vi "RecVOR.vi"() -> ()   [LabVIEW 2013]
uses:
  <vilib>/userdefined/High Color/IMAQdx.ctl
  <vilib>/vision/Avi1.llb/AviRefnum.ctl
  <vilib>/vision/driver/IMAQdx.llb/IMAQdx Attribute Visibility.ctl
  <vilib>/Instr/_visa.llb/VISA Configure Serial Port (Instr).vi
  <vilib>/DAQmx/read.llb/DAQmx Read (Digital Bool 1Line 1Point).vi
  <vilib>/DAQmx/read.llb/DAQmx Read (Counter U32 1Chan 1Samp).vi
  <vilib>/Utility/file.llb/Write To Spreadsheet File (DBL).vi
  <vilib>/vision/driver/NI_Vision_Acquisition_Software.lvlib
  <resource>/objmgr/imaqdx.rc
  <vilib>/vision/NI_Vision_Development_Module.lvlib
panel:
  out "NewRecevie":string
  in  "Use":bool=TRUE
  out "Serial 2":bool
  out "Serial":bool
  in  "Tilting":refnum<visa-resource-name>="COM4"
  in  "Image Flip":u32(ring) items=["Horizontal Flip", "Vertical Flip", "Central Flip", "No Flip"]
  in  "Attribute Name":u32(ring)
  in  "Set":bool
  in  "Attribute Value":string
  in  "Arduino":refnum<visa-resource-name>="COM6"
  out "Pos./Vel.":cluster{dbl, dbl}(graph)
  out "Start RecTime":timestamp
  out "Avi Refnum":T1
  out "Elapsed Time":dbl
  out "Frame Num":dbl
  in  "Codec:":string(combo)="Microsoft Video 1"
  out "Rec File Path:":path
  in  "Recording":bool
  in  "Camera Name:":T2="cam1"
  in  "stop":bool
  in  "OpenCam":bool
  out "Frame Rate":dbl(knob) scale=0.0..120.0
  in  "Tab Control":enum32{"Alignment", "Rotator"}(tab)
  out "Alignment":bool
  in  "BCGT":T3={"Brightness"=171.0, "Contrast"=89.0, "Gamma"=2.0, "Threshold_Low"=0.0, "Threshold_High"=255.0} {"Threshold_High" min=0.0 max=255.0 step=1.0 scale=0.0..255.0; "Threshold_Low" min=0 max=255 step=1 scale=0.0..255.0 scale format="%.2f"; "Gamma" min=0.1 max=10 step=0.01 scale=0.1..10.0 scale format="%.1f"; "Contrast" min=1 max=89 step=0.1 scale=0.0..89.0 scale format="%.2f"; "Brightness" min=0 max=255 step=1 scale=0.0..255.0 scale format="%.2f"}
  out "Number of Particles":i32
  out "Distances":sgl[](array[numeric]) format="%.4f"
  out "Array":cluster{"Numeric":dbl, "Numeric":dbl}[](array[cluster])
  out "Image 2":T4(plugin-control)
  in  "primary":bool
  in  "Clear 2":bool
  in  "Clear":bool
  in  "Tolerence":dbl=90.0
  in  "Add":bool
  in  "mode":enum32{"Sine", "Linear", "Tilting"}(tab)
  in  "Freq":string="0.01" caption="Freq.(Hz)"
  in  "Time":string="10" caption="Operation \nTime(sec)"
  in  "Ang.vel":string="30" caption="Angular\nVelocity\n( ˚/sec)"
  in  "IncT":string="2000" caption="Acceleration\n( ˚/sec²)"
  in  "Ang.vel 2":string="100" caption="Angular\nVelocity\n( ˚/sec)"
  in  "Time 2":string="10" caption="Operation Time(sec)"
  in  "Direction":enum32{"Radio Selection 1", "Radio Selection 2"}(radio)
  out "TiltingLED":bool
  in  "TilAngle":string="30" caption="Tilting\nAngle"
  in  "TilTime":string="2" caption="Tilting\nTime"
  out "ObjAng":dbl
  out "TiltAng.":dbl
  out "WMode":enum16{"stop", "goFront", "goBack"}(ring)
  in  "SeeAngle":bool
  out "check":bool
  out "Degree/sec":dbl(knob) scale=-105.0..105.0
  out "EMST":bool
  out "SVON":bool=TRUE
  out "Received Data":string
  out "Transmit Data":string
  in  "Sent":bool
  in  "task/channels in":refnum<k21>="position"
  in  "task/channels in 2":refnum<k21>="dir"
  in  "task/channels in 3":refnum<k21>="dir_vel"
  out "Angle Position":dbl(knob)
  out "List":string
  in  "StopT":bool
  out "Image":T4(plugin-control)
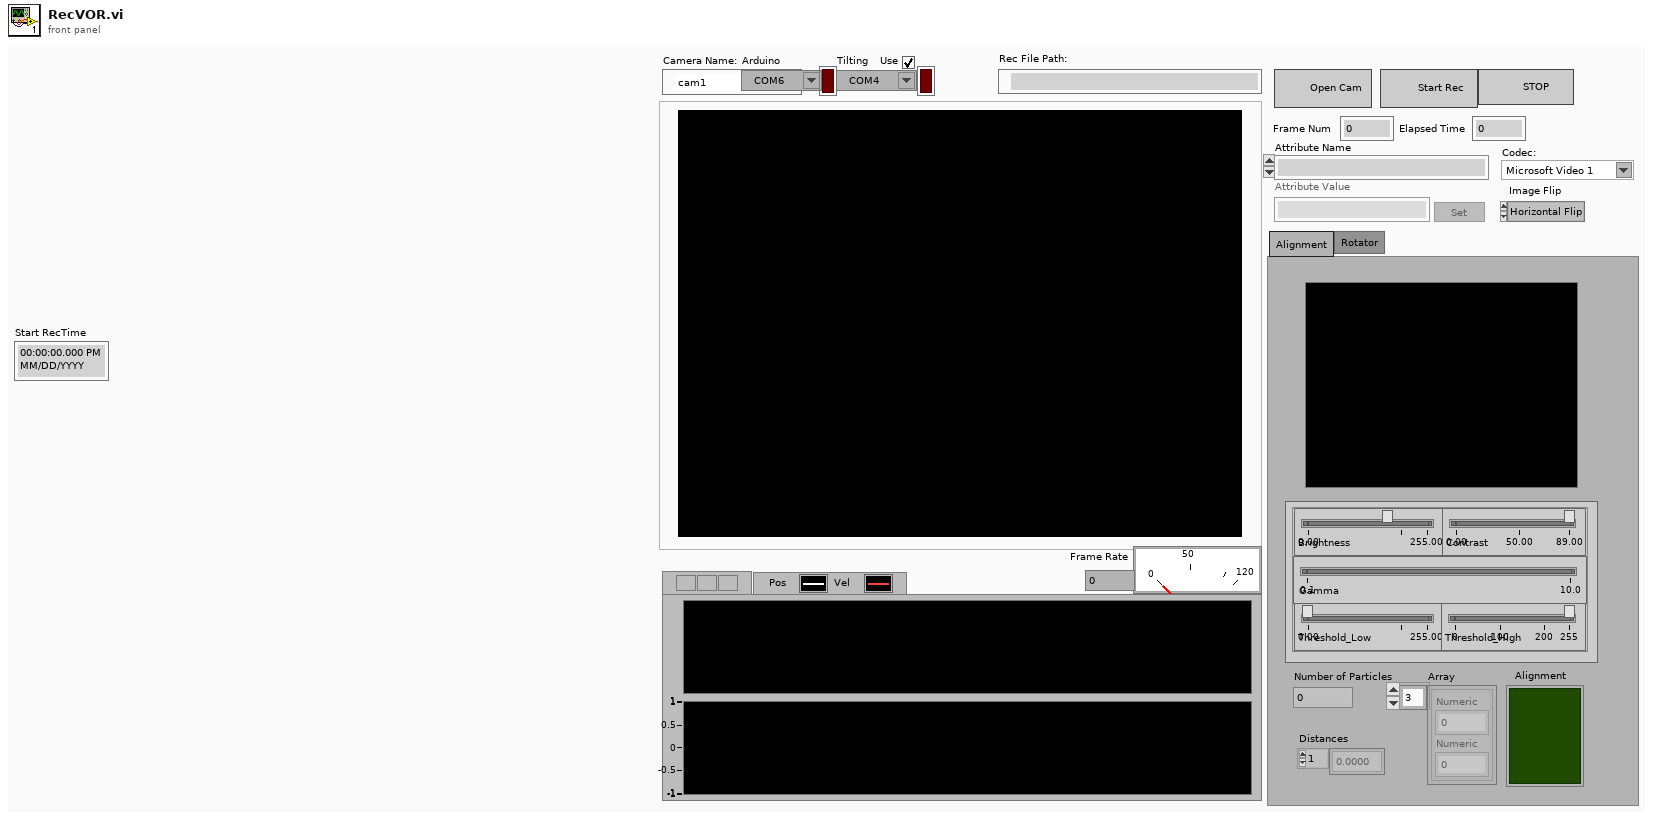
[diagram p1: front panel]
types:
  T1 = typedef "AviRefnum.ctl" = refnum<k1>
  T2 = typedef "IMAQdx.ctl" = refnum<k21>
  T3 = cluster{"Brightness":sgl, "Contrast":sgl, "Gamma":sgl, "Threshold_Low":sgl, "Threshold_High":dbl}
  T4 = typedef "IMAQ Image.ctl" = refnum<image>
  T5 = enum8{"Enabled", "Disabled", "Disabled and Grayed Out"}
  T6 = enum16{"Calvar3Open", "CalDataOpen", "CalGrpOpen", "AddAvg", "RmvAvg", "CalCalvar", "AddVar", "SaveVar", "Up", "Dn", "Del"}
  T7 = enum16{"SVON OFF", "SVON ON", "EMST OFF", "EMST ON", "15 degree, 0.1Hz", "15 degree, 0.2Hz", "15 degree, 0.5Hz", "15 degree, 1Hz", "15 degree, 2Hz", "15 degree, 4Hz", "15 degree, 6Hz", "15 degree, 8Hz", "15 degree, 10Hz", "30 degree, 0.1Hz", "30 degree, 0.2Hz", "30 degree, 0.5Hz", "30 degree, 1Hz", "30 degree, 2Hz", "30 degree, 4Hz", "30 degree, 6Hz", "30 degree, 8Hz", "30 degree, 10Hz", "60 degree, 0.1Hz", "60 degree, 0.2Hz", "60 degree, 0.5Hz", "60 degree, 1Hz", "60 degree, 2Hz", "60 degree, 4Hz", "60 degree, 6Hz", "60 degree, 8Hz", "100 degree, 0.1Hz", "100 degree, 0.2Hz", "100 degree, 0.5Hz", "100 degree, 1Hz"}
  T8 = typedef "NI_Vision_Acquisition_Software.lvlib/IMAQdx Attribute Visibility.ctl" = enum32{"Simple", "Intermediate", "Advanced"}
  T9 = typedef "NI_Vision_Acquisition_Software.lvlib/IMAQdx Attribute Type.ctl" = enum32{"U32", "I64", "DBL", "String", "Enum", "Bool", "Command"}
  T10 = cluster{"Attribute Type":T9, "Readable":bool, "Writable":bool, "Attribute Name":string}[]
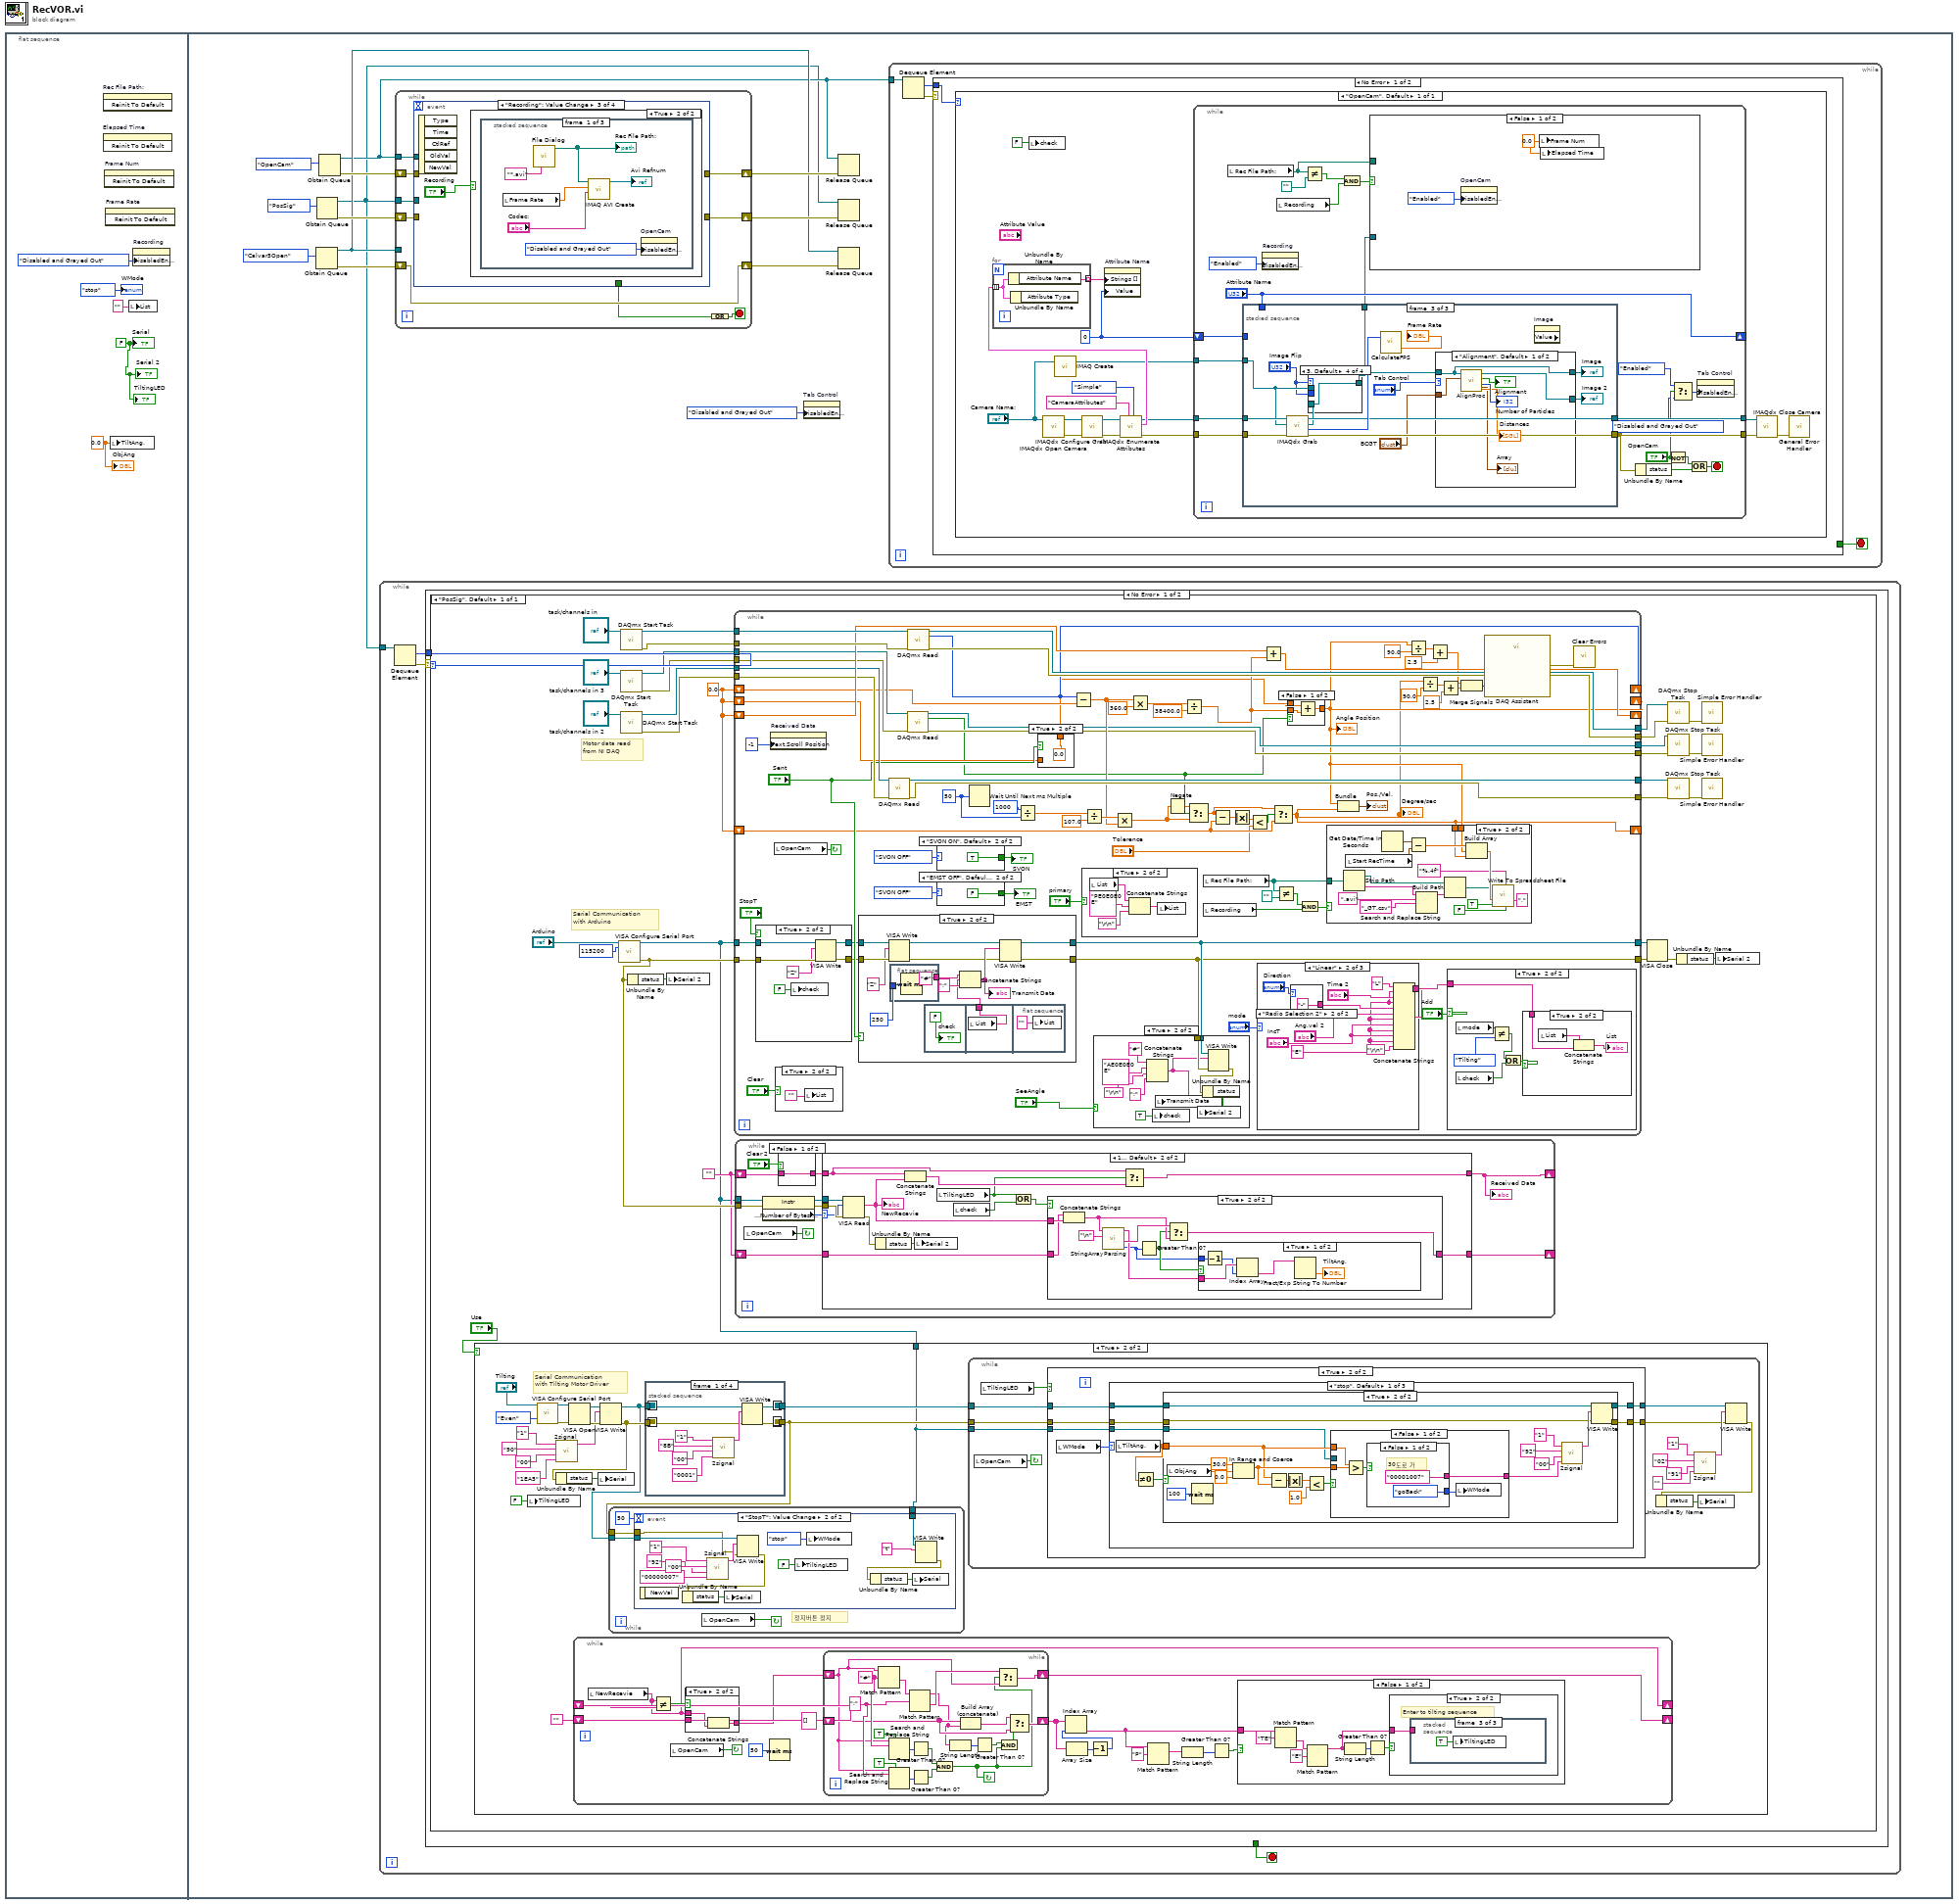
[diagram p0: block diagram]
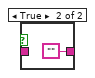
[diagram p2: hidden frame]
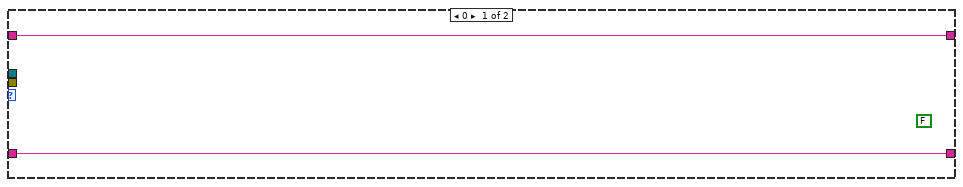
[diagram p3: hidden frame]
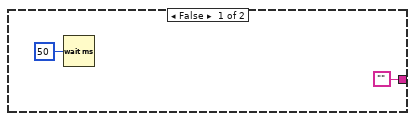
[diagram p4: hidden frame]
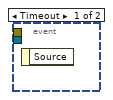
[diagram p7: hidden frame]
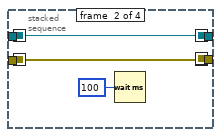
[diagram p8: hidden frame]
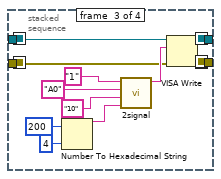
[diagram p9: hidden frame]
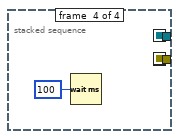
[diagram p10: hidden frame]
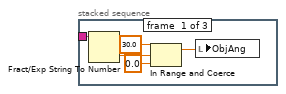
[diagram p12: hidden frame]
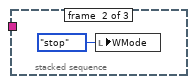
[diagram p13: hidden frame]
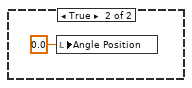
[diagram p14: hidden frame]
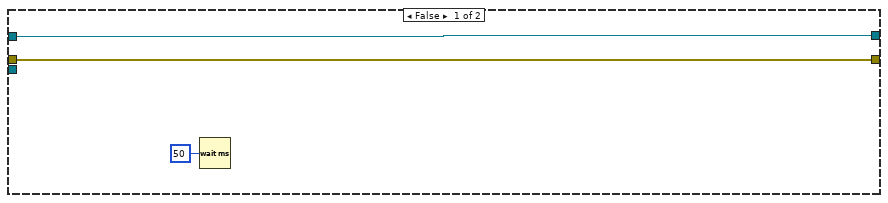
[diagram p16: hidden frame]
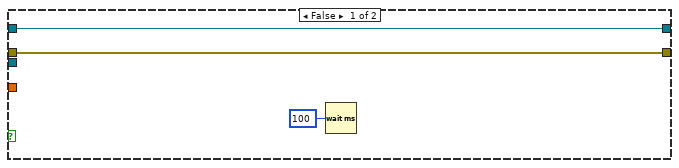
[diagram p17: hidden frame]
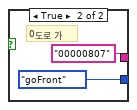
[diagram p18: hidden frame]
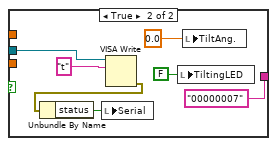
[diagram p19: hidden frame]
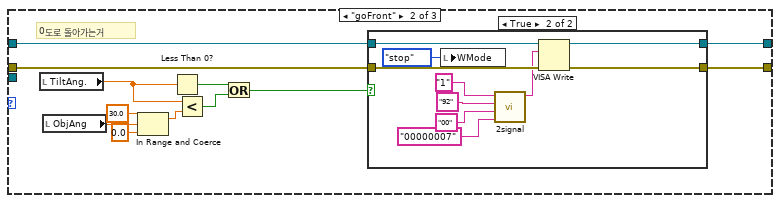
[diagram p20: hidden frame]
diagram:
  n1 = flat-sequence {
    frame #0 {
      w3 = 0.0 ("element")
      w2 = FALSE ("Serial")
      n2 = invoke on="Rec File Path:" class="Path" method="Reinit To Default"() -> ()  [unwired: 3 in, 3 out]
      n3 = invoke on="Elapsed Time" class="DigNum (strict)" method="Reinit To Default"() -> ()  [unwired: 3 in, 3 out]
      n4 = invoke on="Frame Num" class="DigNum (strict)" method="Reinit To Default"() -> ()  [unwired: 3 in, 3 out]
      n5 = invoke on="Frame Rate" class="Knob (strict)" method="Reinit To Default"() -> ()  [unwired: 3 in, 3 out]
      n6 = local write "TiltAng."(w3) -> ()
      n7 = local write "List"("" ("List")) -> ()
      n8 = property on="Recording" class="Bool (strict)"("DisabledEnum"=T5."Disabled and Grayed Out" ("Disabled")) -> ()  [unwired: 2 in, 2 out]
      "Serial" <- w2
      "Serial 2" <- w2
      "ObjAng" <- w3
      "TiltingLED" <- w2
      "WMode" <- enum16{"stop", "goFront", "goBack"}."stop" ("WMode")
    }
    frame #1 {
      n9 = Obtain Queue(element data type=T6."Calvar3Open" ("Enum")) -> (queue out=w9:refnum<queue>, error out=w14:errorcluster)  [unwired: 4 in, 1 out]
      n10 = Obtain Queue(element data type=enum16{"PosSig"}."PosSig" ("Enum")) -> (queue out=w7:refnum<queue>, error out=w15:errorcluster)  [unwired: 4 in, 1 out]
      n11 = Obtain Queue(element data type=enum16{"OpenCam"}."OpenCam" ("Enum")) -> (queue out=w8:refnum<queue>, error out=w17:errorcluster)  [unwired: 4 in, 1 out]
      n12 = while {
        tunnel: w7 -> [w22]
        stop <- w20 stop-if-true
        n13 = Dequeue Element(queue=w22) -> (element=w19:enum16{"PosSig"}, error out=w21:errorcluster)  [unwired: 2 in, 2 out]
        n14 = case shown="No Error" w21 {
          tunnel: [_ TRUE] -> w20
          tunnel: w19 -> [w23 _]
          frame No Error {
            n15 = case shown="\"PosSig\", Default" w23 {
              frame "PosSig", Default {
                w29 = 0.0 ("data")
                w25 = ""
                # "Motor data read\nfrom NI DAQ"
                # "Serial Communication \nwith Arduino"
                n16 = call-poly "VISA Configure Serial Port"("VISA resource name"="Arduino", "baud rate (9600)"=u32 115200) -> ("VISA resource name out"=w24:refnum<visa-resource-name>, "error out"=w28:errorcluster)  [unwired: 12 in]
                n17 = case shown="True" "Use" {
                  tunnel: w24 -> [_ w100]
                  frame False {
                  }
                  frame True {
                    w104 = ""
                    # "Serial Communication\nwith Tilting Motor Driver"
                    n18 = local write "TiltingLED"(FALSE ("TiltingLED")) -> ()
                    n19 = call-poly "VISA Configure Serial Port"("VISA resource name"="Tilting", "parity (0:none)"=enum16{"None", "Odd", "Even", "Mark", "Space"}."Even") -> ("VISA resource name out"=w108:refnum<visa-resource-name>, "error out"=w110:errorcluster)  [unwired: 12 in]
                    n20 = call "2signal.vi"("데이터"="1EA5", "Dat.Num"="00", "커맨드"="90", "국번"="1") -> ("String"=w107:string)  [unwired: 7 in]
                    n21 = VISA Open(error in (no error)=w110, VISA resource name=w108) -> (VISA resource name=w113:refnum<visa-resource-name>, error out=w112:errorcluster)  [unwired: 3 in]
                    n22 = while {
                      shift-right: [w175] -> _
                      shift-left: w104 -> [w176]
                      shift-right: [w170] -> _
                      shift-left: w104 -> [w172]
                      stop <- w173 continue-if-true
                      n23 = local read "NewRecevie"() -> (w170:string)
                      n24 = Not Equal?(x=w170, y=w172) -> (x != y?=w171:bool)
                      n25 = local read "OpenCam"() -> (w173:bool)
                      n26 = case shown="True" w171 {
                        tunnel: w176 -> [w218 w221]
                        tunnel: [w218 w220] -> w180
                        tunnel: w170 -> [_ w219]
                        frame False {
                        }
                        frame True {
                          n27 = Concatenate Strings(w221, w219) -> (w220:string)
                        }
                      }
                      n28 = Wait (ms)(milliseconds to wait=u32 50) -> ()  [unwired: 1 out]
                      n29 = while {
                        shift-right: [w205] -> w177
                        shift-left: string[] [] -> [w203]
                        shift-right: [w208] -> w175
                        shift-left: w180 -> [w206]
                        stop <- w199 continue-if-true
                        w213 = ";" ("regular expression")
                        w215 = "#" ("regular expression")
                        n30 = Match Pattern(string=w206, regular expression=w215) -> (after substring=w217:string)  [unwired: 1 in, 3 out]
                        n31 = Search and Replace String(replace all?=TRUE ("replace all? (F)"), input string=w206, search string=w215) -> (number of replacements=w212:i32)  [unwired: 5 in, 3 out]
                        n32 = Search and Replace String(replace all?=TRUE ("replace all? (F)"), input string=w206, search string=w213) -> (number of replacements=w211:i32)  [unwired: 5 in, 3 out]
                        n33 = Match Pattern(string=w217, regular expression=w213) -> (before substring=w202:string, after substring=w207:string)  [unwired: 1 in, 2 out]
                        n34 = Greater Than 0?(x=w212) -> (x > 0?=w209:bool)
                        n35 = Greater Than 0?(x=w211) -> (x > 0?=w210:bool)
                        n36 = And(x=w209, y=w210) -> (x .and. y?=w199:bool)
                        n37 = String Length(string=w202) -> (length=w201:i32)
                        n38 = Build Array (concatenate)(w203, w202) -> (w204:string[])
                        n39 = Greater Than 0?(x=w201) -> (x > 0?=w200:bool)
                        n40 = Select(t=w207, s=w199, f=w206) -> (s? t:f=w208:string)
                        n41 = And(x=w200, y=w199) -> (x .and. y?=w198:bool)
                        n42 = Select(t=w204, s=w198, f=w203) -> (s? t:f=w205:string[])
                      }
                      n43 = Array Size(array=w177) -> (size(s)=w178:i32)
                      n44 = Decrement(x=w178) -> (x-1=w179:i32)
                      n45 = Index Array(array=w177, index=w179) -> (element=w168:string)
                      n46 = Match Pattern(string=w168, regular expression="P") -> (match substring=w165:string)  [unwired: 1 in, 3 out]
                      n47 = String Length(string=w165) -> (length=w167:i32)
                      n48 = Greater Than 0?(x=w167) -> (x > 0?=w166:bool)
                      n49 = case shown="False" w166 {
                        tunnel: w168 -> [w188 _]
                        frame False {
                          n50 = Match Pattern(string=w188, regular expression="TE") -> (after substring=w185:string)  [unwired: 1 in, 3 out]
                          n51 = Match Pattern(string=w185, regular expression="E") -> (before substring=w182:string)  [unwired: 1 in, 3 out]
                          n52 = String Length(string=w182) -> (length=w184:i32)
                          n53 = Greater Than 0?(x=w184) -> (x > 0?=w183:bool)
                          n54 = case shown="True" w183 {
                            tunnel: w182 -> [_ w189]
                            frame False {
                            }
                            frame True {
                              # "Enter to tilting sequence"
                              n55 = stacked-sequence {
                                tunnel: w189 -> [w194 _ _]
                                frame #0 {
                                n56 = Fract/Exp String To Number(string=w194) -> (number=w193:dbl)  [unwired: 3 in, 1 out]
                                n57 = In Range and Coerce(upper limit=30.0, x=w193, lower limit=0.0) -> (coerced(x)=w192:dbl)  [unwired: 1 out]
                                n58 = local write "ObjAng"(w192) -> ()
                                }
                                frame #1 {
                                n59 = local write "WMode"(enum16{"stop", "goFront", "goBack"}."stop" ("WMode")) -> ()
                                }
                                frame #2 {
                                n60 = local write "TiltingLED"(TRUE ("TiltingLED")) -> ()
                                }
                              }
                            }
                          }
                        }
                        frame True {
                          n61 = local write "Angle Position"(0.0 ("Angle Position")) -> ()
                        }
                      }
                    }
                    n62 = VISA Write(VISA resource name=w113, write buffer=w107, error in (no error)=w112) -> (VISA resource name out=w102:refnum<visa-resource-name>, error out=w106:errorcluster)  [unwired: 1 out]
                    n63 = Unbundle By Name(w106) -> ("status"=w118:bool)
                    n64 = local write "Serial"(w118) -> ()
                    n65 = stacked-sequence {
                      seq-local: [w140 _ _ _] -> [_ w149 _ _]
                      seq-local: [w139 _ _ _] -> [_ w148 _ _]
                      seq-local: [_ w149 _ _] -> [_ _ w155 _]
                      seq-local: [_ w148 _ _] -> [_ _ w154 _]
                      seq-local: [_ _ w152 _] -> [_ _ _ w163]
                      seq-local: [_ _ w151 _] -> [_ _ _ w162]
                      tunnel: w102 -> [w142 _ _ _]
                      tunnel: w106 -> [w141 _ _ _]
                      tunnel: [_ _ _ w163] -> w105
                      tunnel: [_ _ _ w162] -> w101
                      frame #0 {
                        n66 = call "2signal.vi"("데이터"="0001", "Dat.Num"="00", "커맨드"="8B", "국번"="1") -> ("String"=w143:string)  [unwired: 7 in]
                        n67 = VISA Write(VISA resource name=w142, write buffer=w143, error in (no error)=w141) -> (VISA resource name out=w140:refnum<visa-resource-name>, error out=w139:errorcluster)  [unwired: 1 out]
                      }
                      frame #1 {
                        n68 = Wait (ms)(milliseconds to wait=u32 100) -> ()  [unwired: 1 out]
                      }
                      frame #2 {
                        n69 = Number To Hexadecimal String(1:i16 4 ("width (-)"), 2:200 ("number")) -> (0:w156:string)
                        n70 = call "2signal.vi"("데이터"=w156, "Dat.Num"="10", "커맨드"="A0", "국번"="1") -> ("String"=w161:string)  [unwired: 7 in]
                        n71 = VISA Write(VISA resource name=w155, write buffer=w161, error in (no error)=w154) -> (VISA resource name out=w152:refnum<visa-resource-name>, error out=w151:errorcluster)  [unwired: 1 out]
                      }
                      frame #3 {
                        n72 = Wait (ms)(milliseconds to wait=u32 100) -> ()  [unwired: 1 out]
                      }
                    }
                    n73 = while {
                      tunnel: w102 -> [w122]
                      tunnel: w101 -> [w121]
                      tunnel: w100 -> [w119]
                      stop <- w120 continue-if-true
                      # "정지버튼 정지"
                      n74 = event shown="[1] \"StopT\": Value Change" {
                        selector: _ -> [_ _]
                        dyn-events: _ -> [_ _]
                        timeout: 50 -> [_ _]
                        tunnel: w122 -> [_ w131]
                        tunnel: w121 -> [_ w130]
                        tunnel: w119 -> [_ w124]
                        event Timeout {
                          n75 = event-data() -> ()  [unwired: 1 in, 1 out]
                        }
                        event "StopT": Value Change {
                          n76 = event-data() -> ()  [unwired: 1 in, 1 out]
                          n77 = call "2signal.vi"("데이터"="00000007", "Dat.Num"="00", "커맨드"="92", "국번"="1") -> ("String"=w134:string)  [unwired: 7 in]
                          n78 = VISA Write(VISA resource name=w131, write buffer=w134, error in (no error)=w130) -> (error out=w132:errorcluster)  [unwired: 2 out]
                          n79 = Unbundle By Name(w132) -> ("status"=w133:bool)
                          n80 = local write "Serial"(w133) -> ()
                          n81 = local write "TiltingLED"(FALSE ("TiltingLED")) -> ()
                          n82 = local write "WMode"(enum16{"stop", "goFront", "goBack"}."stop" ("WMode")) -> ()
                          n83 = VISA Write(VISA resource name=w124, write buffer="t") -> (error out=w125:errorcluster)  [unwired: 1 in, 2 out]
                          n84 = Unbundle By Name(w125) -> ("status"=w127:bool)
                          n85 = local write "Serial"(w127) -> ()
                        }
                      }
                      n86 = local read "OpenCam"() -> (w120:bool)
                    }
                    n87 = while {
                      tunnel: w105 -> [w226]
                      tunnel: w101 -> [w223]
                      tunnel: w100 -> [w222]
                      stop <- w235 continue-if-true
                      n88 = local read "OpenCam"() -> (w235:bool)
                      n89 = local read "TiltingLED"() -> (w227:bool)
                      n90 = case shown="True" w227 {
                        tunnel: w226 -> [w238 w244]
                        tunnel: w223 -> [w237 w243]
                        tunnel: [w238 w242] -> w229
                        tunnel: [w237 w241] -> w228
                        tunnel: w222 -> [_ w239]
                        frame False {
                          n91 = Wait (ms)(milliseconds to wait=u32 50) -> ()  [unwired: 1 out]
                        }
                        frame True {
                          n92 = local read "WMode"() -> (w240:enum16{"stop", "goFront", "goBack"})
                          n93 = case shown="\"stop\", Default" w240 {
                            tunnel: w244 -> [w251 w302 w326]
                            tunnel: w243 -> [w250 w301 w325]
                            tunnel: [w248 w299 w323] -> w242
                            tunnel: [w249 w300 w324] -> w241
                            tunnel: w239 -> [w247 _ _]
                            frame "stop", Default {
                              n94 = local read "TiltAng."() -> (w246:dbl)
                              n95 = Not Equal To 0?(x=w246) -> (x != 0?=w245:bool)
                              n96 = case shown="True" w245 {
                                tunnel: w251 -> [w254 w271]
                                tunnel: w250 -> [w253 w270]
                                tunnel: [w253 w268] -> w249
                                tunnel: [w254 w267] -> w248
                                tunnel: w246 -> [_ w257]
                                tunnel: w247 -> [_ w255]
                                frame False {
                                n97 = Wait (ms)(milliseconds to wait=u32 100) -> ()  [unwired: 1 out]
                                }
                                frame True {
                                n98 = local read "ObjAng"() -> (w263:dbl)
                                n99 = Wait (ms)(milliseconds to wait=u32 100) -> ()  [unwired: 1 out]
                                n100 = In Range and Coerce(upper limit=30.0, x=w263, lower limit=0.0) -> (coerced(x)=w261:dbl)  [unwired: 1 out]
                                n101 = Subtract(x=w257, y=w261) -> (x-y=w260:dbl)
                                n102 = Absolute Value(x=w260) -> (abs(x)=w259:dbl)
                                n103 = Less?(x=w259, y=1.0) -> (x < y?=w256:bool)
                                n104 = case shown="False" w256 {
                                tunnel: [w279 "00000007"] -> w266
                                tunnel: w257 -> [w276 _]
                                tunnel: w261 -> [w275 _]
                                tunnel: w255 -> [_ w285]
                                frame False {
                                n105 = Greater?(x=w276, y=w275) -> (0:w277:bool)
                                n106 = case shown="False" w277 {
                                tunnel: ["00001007" "00000807"] -> w279
                                tunnel: [enum16{"stop", "goFront", "goBack"}."goBack" ("WMode") enum16{"stop", "goFront", "goBack"}."goFront" ("WMode")] -> w278
                                frame False {
                                # "30도로 가"
                                }
                                frame True {
                                # "0도로 가"
                                }
                                }
                                n107 = local write "WMode"(w278) -> ()
                                }
                                frame True {
                                n108 = VISA Write(VISA resource name=w285, write buffer="t") -> (error out=w286:errorcluster)  [unwired: 1 in, 2 out]
                                n109 = Unbundle By Name(w286) -> ("status"=w287:bool)
                                n110 = local write "Serial"(w287) -> ()
                                n111 = local write "TiltingLED"(FALSE ("TiltingLED")) -> ()
                                n112 = local write "TiltAng."(0.0 ("lower limit")) -> ()
                                }
                                }
                                n113 = call "2signal.vi"("데이터"=w266, "Dat.Num"="00", "커맨드"="92", "국번"="1") -> ("String"=w272:string)  [unwired: 7 in]
                                n114 = VISA Write(VISA resource name=w271, write buffer=w272, error in (no error)=w270) -> (VISA resource name out=w267:refnum<visa-resource-name>, error out=w268:errorcluster)  [unwired: 1 out]
                                }
                              }
                            }
                            frame "goFront" {
                              # "0도로 돌아가는거"
                              n115 = local read "TiltAng."() -> (w292:dbl)
                              n116 = local read "ObjAng"() -> (w295:dbl)
                              n117 = In Range and Coerce(upper limit=30.0, x=w295, lower limit=0.0) -> (coerced(x)=w294:dbl)  [unwired: 1 out]
                              n118 = Less Than 0?(x=w292) -> (x < 0?=w291:bool)
                              n119 = Less?(x=w292, y=w294) -> (x < y?=w293:bool)
                              n120 = Or(x=w291, y=w293) -> (x .or. y?=w298:bool)
                              n121 = case shown="True" w298 {
                                tunnel: w302 -> [w304 w314]
                                tunnel: w301 -> [w303 w313]
                                tunnel: [w303 w305] -> w300
                                tunnel: [w304 w312] -> w299
                                frame False {
                                }
                                frame True {
                                n122 = local write "WMode"(enum16{"stop", "goFront", "goBack"}."stop" ("WMode")) -> ()
                                n123 = call "2signal.vi"("데이터"="00000007", "Dat.Num"="00", "커맨드"="92", "국번"="1") -> ("String"=w307:string)  [unwired: 7 in]
                                n124 = VISA Write(VISA resource name=w314, write buffer=w307, error in (no error)=w313) -> (VISA resource name out=w312:refnum<visa-resource-name>, error out=w305:errorcluster)  [unwired: 1 out]
                                }
                              }
                            }
                            frame "goBack" {
                              w316 = 30.0 ("upper limit")
                              # "30도로 기울어지는거"
                              n125 = local read "ObjAng"() -> (w320:dbl)
                              n126 = local read "TiltAng."() -> (w317:dbl)
                              n127 = In Range and Coerce(upper limit=w316, x=w320, lower limit=0.0) -> (coerced(x)=w321:dbl)  [unwired: 1 out]
                              n128 = Less?(x=w316, y=w317) -> (x < y?=w315:bool)
                              n129 = Greater?(x=w317, y=w321) -> (0:w322:bool)
                              n130 = Or(x=w315, y=w322) -> (x .or. y?=w318:bool)
                              n131 = case shown="True" w318 {
                                tunnel: w326 -> [w328 w338]
                                tunnel: w325 -> [w327 w337]
                                tunnel: [w327 w336] -> w324
                                tunnel: [w328 w335] -> w323
                                frame False {
                                }
                                frame True {
                                n132 = local write "WMode"(enum16{"stop", "goFront", "goBack"}."stop" ("WMode")) -> ()
                                n133 = call "2signal.vi"("데이터"="00000007", "Dat.Num"="00", "커맨드"="92", "국번"="1") -> ("String"=w330:string)  [unwired: 7 in]
                                n134 = VISA Write(VISA resource name=w338, write buffer=w330, error in (no error)=w337) -> (VISA resource name out=w335:refnum<visa-resource-name>, error out=w336:errorcluster)  [unwired: 1 out]
                                }
                              }
                            }
                          }
                        }
                      }
                      n135 = call "2signal.vi"("데이터"="", "Dat.Num"="91", "커맨드"="02", "국번"="1") -> ("String"=w234:string)  [unwired: 7 in]
                      n136 = VISA Write(VISA resource name=w229, write buffer=w234, error in (no error)=w228) -> (error out=w224:errorcluster)  [unwired: 2 out]
                      n137 = Unbundle By Name(w224) -> ("status"=w225:bool)
                      n138 = local write "Serial"(w225) -> ()
                    }
                  }
                }
                n139 = call <vilib>:"DAQmx Start Task.vi"("task/channels in"="task/channels in") -> ("task out"=w49:refnum<k21>, "error out"=w46:errorcluster)  [unwired: 13 in]
                n140 = call <vilib>:"DAQmx Start Task.vi"("task/channels in"="task/channels in 3") -> ("task out"=w37:refnum<k21>, "error out"=w36:errorcluster)  [unwired: 13 in]
                n141 = call <vilib>:"DAQmx Start Task.vi"("task/channels in"="task/channels in 2") -> ("task out"=w43:refnum<k21>, "error out"=w42:errorcluster)  [unwired: 13 in]
                n142 = Unbundle By Name(w28) -> ("status"=w31:bool)
                n143 = local write "Serial 2"(w31) -> ()
                n144 = while {
                  tunnel: w28 -> [w355]
                  tunnel: w24 -> [w356]
                  tunnel: [w339] -> w52
                  tunnel: [w340] -> w53
                  tunnel: [w411] -> w50
                  tunnel: w49 -> [w410]
                  tunnel: w46 -> [w409]
                  tunnel: [w408] -> w48
                  shift-right: [w399] -> _
                  shift-left: w29 -> [w385]
                  shift-right: [w398] -> _
                  shift-left: w29 -> [w404]
                  tunnel: w43 -> [w403]
                  tunnel: w42 -> [w402]
                  tunnel: [w401] -> w41
                  tunnel: [w400] -> w40
                  shift-right: [w353] -> _
                  shift-left: w29 -> [w384]
                  tunnel: w37 -> [w390]
                  tunnel: w36 -> [w389]
                  tunnel: [w388] -> w34
                  tunnel: [w387] -> w33
                  shift-right: [w347] -> _
                  shift-left: w29 -> [w366]
                  stop <- w362 continue-if-true
                  w397 = u32 50 ("millisecond multiple")
                  n145 = case shown="True" "StopT" {
                    tunnel: [w429 w435] -> w359
                    tunnel: w356 -> [w429 w433]
                    tunnel: [w428 w434] -> w358
                    tunnel: w355 -> [w428 w432]
                    frame False {
                    }
                    frame True {
                      n146 = local write "check"(FALSE ("check")) -> ()
                      n147 = VISA Write(VISA resource name=w433, write buffer="Z", error in (no error)=w432) -> (VISA resource name out=w435:refnum<visa-resource-name>, error out=w434:errorcluster)  [unwired: 1 out]
                    }
                  }
                  n148 = property on="Received Data" class="Str"("Text.Scroll Position"=-1) -> ()  [unwired: 2 in, 2 out]
                  n149 = local read "OpenCam"() -> (w362:bool)
                  n150 = case shown="True" "Clear" {
                    frame False {
                    }
                    frame True {
                      n151 = local write "List"("") -> ()
                    }
                  }
                  n152 = case shown="True" "Sent" {
                    tunnel: w359 -> [w501 w507]
                    tunnel: w358 -> [w500 w506]
                    tunnel: [w501 w513] -> w340
                    tunnel: [w500 w512] -> w339
                    frame False {
                    }
                    frame True {
                      n153 = VISA Write(VISA resource name=w507, write buffer="Z", error in (no error)=w506) -> (VISA resource name out=w504:refnum<visa-resource-name>, error out=w503:errorcluster)  [unwired: 1 out]
                      n154 = flat-sequence {
                        tunnel: ["#"] -> w510
                        tunnel: u32 250 ("millisecond multiple") -> [w514]
                        frame #0 {
                          n155 = Wait (ms)(milliseconds to wait=w514) -> ()  [unwired: 1 out]
                        }
                      }
                      n156 = flat-sequence {
                        tunnel: [w517] -> w508
                        frame #0 {
                          "check" <- FALSE
                        }
                        frame #1 {
                          n157 = local read "List"() -> (w517:string)
                        }
                        frame #2 {
                          n158 = local write "List"("" ("List")) -> ()
                        }
                      }
                      n159 = Concatenate Strings(w510, w508, ";") -> (w509:string)
                      "Transmit Data" <- w509
                      n160 = VISA Write(VISA resource name=w504, write buffer=w509, error in (no error)=w503) -> (VISA resource name out=w513:refnum<visa-resource-name>, error out=w512:errorcluster)  [unwired: 1 out]
                    }
                  }
                  n161 = call-poly <vilib>:"DAQmx Read.vi"("task/channels in"=w403, "error in"=w402) -> ("task out"=w400:refnum<k21>, "error out"=w401:errorcluster)  [unwired: 11 in, 1 out]
                  n162 = call-poly <vilib>:"DAQmx Read.vi"("task/channels in"=w390, "error in"=w389) -> ("task out"=w387:refnum<k21>, "data"=w367:bool, "error out"=w388:errorcluster)  [unwired: 11 in]
                  n163 = call-poly <vilib>:"DAQmx Read.vi"("task/channels in"=w410, "error in"=w409) -> ("task out"=w408:refnum<k21>, "data"=w399:u32, "error out"=w411:errorcluster)  [unwired: 11 in]
                  n164 = case shown="\"SVON ON\", Default" T7."SVON OFF" ("Select Mode") {
                    tunnel: [FALSE TRUE] -> w413
                    frame "SVON OFF" {
                    }
                    frame "SVON ON", Default {
                    }
                  }
                  "SVON" <- w413
                  n165 = case shown="\"EMST OFF\", Default" T7."SVON OFF" ("Select Mode") {
                    tunnel: [TRUE FALSE] -> w412
                    frame "EMST ON" {
                    }
                    frame "EMST OFF", Default {
                    }
                  }
                  "EMST" <- w412
                  n166 = Wait Until Next ms Multiple(millisecond multiple=w397) -> ()  [unwired: 1 out]
                  n167 = Divide(x=u32 1000, y=w397) -> (x/y=w391:dbl)
                  n168 = case shown="True" "Sent" {
                    tunnel: w384 -> [w488 _]
                    tunnel: [w488 0.0] -> w383
                    frame False {
                    }
                    frame True {
                    }
                  }
                  n169 = Subtract(x=w399, y=w385) -> (x-y=w393:dbl)
                  n170 = case shown="True" "primary" {
                    frame False {
                    }
                    frame True {
                      n171 = local read "List"() -> (w425:string)
                      n172 = Concatenate Strings(w425, "PE0E0E0E" ("string"), "\r\n") -> (w424:string)
                      n173 = local write "List"(w424) -> ()
                    }
                  }
                  n174 = Divide(x=w391, y=107.0 ("x")) -> (x/y=w395:dbl)
                  n175 = case shown="True" "SeeAngle" {
                    tunnel: w340 -> [_ w423]
                    tunnel: w339 -> [_ w422]
                    frame False {
                    }
                    frame True {
                      n176 = Concatenate Strings("#", "AE0E0E0E" ("string"), "\r\n", ";") -> (w414:string)
                      n177 = local write "check"(TRUE ("check")) -> ()
                      n178 = local write "Transmit Data"(w414) -> ()
                      n179 = VISA Write(VISA resource name=w423, write buffer=w414, error in (no error)=w422) -> (error out=w420:errorcluster)  [unwired: 2 out]
                      n180 = Unbundle By Name(w420) -> ("status"=w421:bool)
                      n181 = local write "Serial 2"(w421) -> ()
                    }
                  }
                  n182 = Multiply(x=w395, y=w393) -> (x*y=w368:dbl)
                  n183 = Multiply(x=w393, y=360.0) -> (x*y=w406:dbl)
                  n184 = Negate(x=w368) -> (-x=w373:dbl)
                  n185 = Divide(x=w406, y=38400.0) -> (x/y=w394:dbl)
                  n186 = Select(t=w373, s=w367, f=w368) -> (s? t:f=w369:dbl)
                  n187 = local read "Rec File Path:"() -> (w378:path)
                  n188 = local read "Recording"() -> (w361:bool)
                  n189 = Subtract(x=w369, y=w366) -> (x-y=w372:dbl)
                  n190 = Absolute Value(x=w372) -> (abs(x)=w370:dbl)
                  n191 = Less?(x=w370, y="Tolerence") -> (x < y?=w371:bool)
                  n192 = case shown="\"Linear\"" "mode" {
                    tunnel: [w453 w462 w465] -> w363
                    frame "Sine", Default {
                      w447 = "E"
                      n193 = Concatenate Strings("S", w447, "Time", w447, "Ang.vel", w447, "Freq", w447, "\r\n") -> (w453:string)
                    }
                    frame "Linear" {
                      w455 = "E"
                      n194 = case shown="\"Radio Selection 2\"" "Direction" {
                        tunnel: ["" "-"] -> w458
                        frame "Radio Selection 1", Default {
                        }
                        frame "Radio Selection 2" {
                        }
                      }
                      n195 = Concatenate Strings("L", w455, "Time 2", w455, w458, "Ang.vel 2", w455, "IncT", w455, "IncT", w455, "\r\n") -> (w462:string)
                    }
                    frame "Tilting" {
                      w469 = "E"
                      n196 = Concatenate Strings("T", w469, "TilAngle", w469, "TilTime", w469, "\r\n") -> (w465:string)
                    }
                  }
                  n197 = Add(x=w404, y=w394) -> (x+y=w398:dbl)
                  n198 = Select(t=w369, s=w371, f=w366) -> (s? t:f=w347:dbl)
                  "Degree/sec" <- w347
                  n199 = Not Equal?(x=w378, y=path "") -> (x != y?=w380:bool)
                  n200 = case shown="False" w367 {
                    tunnel: w394 -> [w492 w494]
                    tunnel: [w491 w493] -> w353
                    tunnel: w383 -> [w490 w495]
                    frame False {
                      n201 = Add(x=w490, y=w492) -> (x+y=w491:dbl)
                    }
                    frame True {
                      n202 = Subtract(x=w495, y=w494) -> (x-y=w493:dbl)
                    }
                  }
                  "Angle Position" <- w353
                  n203 = And(x=w380, y=w361) -> (x .and. y?=w379:bool)
                  n204 = case shown="True" w379 {
                    tunnel: w353 -> [_ w481]
                    tunnel: w347 -> [_ w480]
                    tunnel: w378 -> [_ w472]
                    frame False {
                    }
                    frame True {
                      n205 = Strip Path(path=w472) -> (stripped path=w474:path, name=w475:string)
                      n206 = local read "Start RecTime"() -> (w487:timestamp)
                      n207 = Get Date/Time In Seconds() -> (seconds since 1Jan1904=w486:timestamp)
                      n208 = Subtract(x=w486, y=w487) -> (x-y=w482:dbl)
                      n209 = Search and Replace String(input string=w475, search string=".avi", replace string="_GT.csv" ("replace string (\"\")")) -> (result string=w478:string)  [unwired: 5 in, 3 out]
                      n210 = Build Path(base path=w474, name or relative path=w478) -> (appended path=w473:path)
                      n211 = Build Array(w482, w481, w480) -> (w479:dbl[])
                      n212 = call-poly <vilib>:"Write To Spreadsheet File.vi"("delimiter (\\t)"="," ("delimiter (\\t)"), "transpose? (no:F)"=FALSE, "format (%.3f)"="%.4f", "append to file? (new file:F)"=TRUE, "1D data"=w479, "file path (dialog if empty)"=w473) -> ()  [unwired: 2 in, 1 out]
                    }
                  }
                  n213 = Bundle(w353, "data"=w347) -> (→"Pos./Vel.":cluster{dbl, "data":dbl})  [unwired: 1 in]
                  n214 = Divide(x=w353, y=90.0) -> (x/y=w351:dbl)
                  n215 = Divide(x=w347, y=90.0) -> (x/y=w349:dbl)
                  n216 = Add(x=w351, y=2.5) -> (x+y=w345:dbl)
                  n217 = Add(x=w349, y=2.5) -> (x+y=w346:dbl)
                  n218 = case shown="True" "Add" {
                    tunnel: w363 -> [_ w437]
                    frame False {
                    }
                    frame True {
                      n219 = local read "mode"() -> (w442:enum32{"Sine", "Linear", "Tilting"})
                      n220 = local read "check"() -> (w440:bool)
                      n221 = Not Equal?(x=w442, y=enum32{"Sine", "Linear", "Tilting"}."Tilting" ("mode")) -> (x != y?=w438:bool)
                      n222 = Or(x=w438, y=w440) -> (x .or. y?=w439:bool)
                      n223 = case shown="True" w439 {
                        tunnel: w437 -> [_ w444]
                        frame False {
                          n224 = One Button Dialog(message="Please check the angle." ("string")) -> ()  [unwired: 1 in, 1 out]
                        }
                        frame True {
                          n225 = local read "List"() -> (w446:string)
                          n226 = Concatenate Strings(w446, w444) -> (→"List":string)
                        }
                      }
                    }
                  }
                  n227 = Merge Signals(w345, w346) -> (w354:dynamicdata)
                  n228 = call "DAQ Assistant"("data"=w354) -> ("error out"=w343:errorcluster)  [unwired: 17 in, 1 out]
                  n229 = call <vilib>:"Clear Errors.vi"("error in (no error)"=w343) -> ()  [unwired: 6 in, 1 out]
                }
                n230 = while {
                  shift-right: [w56] -> _
                  shift-left: w25 -> [w60]
                  tunnel: w24 -> [w59]
                  tunnel: w28 -> [w58]
                  shift-right: [w55] -> _
                  shift-left: w25 -> [w54]
                  stop <- w62 continue-if-true
                  n231 = local read "OpenCam"() -> (w62:bool)
                  n232 = property class="Instr"(reference=w59, error in=w58) -> (reference out=w63:refnum<visa-resource-name>, error out=w64:errorcluster, "Serial Settings:Number of Bytes at Serial Port"=w65:u32)
                  n233 = case shown="False" "Clear 2" {
                    tunnel: w60 -> [w66 _]
                    tunnel: [w66 ""] -> w57
                    frame False {
                    }
                    frame True {
                    }
                  }
                  n234 = case shown="1.., Default" w65 {
                    selector: w65 -> [_ w81]
                    tunnel: w64 -> [_ w83]
                    tunnel: w63 -> [_ w82]
                    tunnel: w57 -> [w69 w80]
                    tunnel: [w69 w79] -> w56
                    tunnel: [w68 w75] -> w55
                    tunnel: w54 -> [w68 w73]
                    frame 0 {
                      (unwired) FALSE ("Read")
                    }
                    frame 1.., Default {
                      n235 = VISA Read(VISA resource name=w82, byte count=w81, error in (no error)=w83) -> (read buffer=w74:string, error out=w76:errorcluster)  [unwired: 2 out]
                      "NewRecevie" <- w74
                      n236 = Unbundle By Name(w76) -> ("status"=w77:bool)
                      n237 = Concatenate Strings(w80, w74) -> (w78:string)
                      n238 = local write "Serial 2"(w77) -> ()
                      n239 = local read "TiltingLED"() -> (w72:bool)
                      n240 = local read "check"() -> (w70:bool)
                      n241 = Or(x=w72, y=w70) -> (x .or. y?=w71:bool)
                      n242 = case shown="True" w71 {
                        tunnel: ["" w91] -> w75
                        tunnel: w74 -> [_ w94]
                        tunnel: w73 -> [_ w86]
                        frame False {
                          n243 = Wait (ms)(milliseconds to wait=u32 50) -> ()  [unwired: 1 out]
                        }
                        frame True {
                          n244 = Concatenate Strings(w86, w94) -> (w92:string)
                          n245 = call "StringArrayParsing.vi"("delimiter"="\n", "Input String"=w92) -> ("#ofPerfectElement"=w88:i32, "After"=w93:string, "Result"=w89:string[])  [unwired: 5 in, 1 out]
                          n246 = Greater Than 0?(x=w88) -> (x > 0?=w90:bool)
                          n247 = Select(t=w93, s=w90, f=w92) -> (s? t:f=w91:string)
                          n248 = case shown="True" w90 {
                            tunnel: w89 -> [w99 _]
                            tunnel: w88 -> [w98 _]
                            frame True {
                              n249 = Decrement(x=w98) -> (x-1=w97:i32)
                              n250 = Index Array(array=w99, index=w97) -> (element=w96:string)
                              n251 = Fract/Exp String To Number(string=w96) -> (number=→"TiltAng.":dbl)  [unwired: 3 in, 1 out]
                            }
                            frame False {
                            }
                          }
                        }
                      }
                      n252 = Select(t=w80, s=w72, f=w78) -> (s? t:f=w79:string)
                    }
                  }
                  "Received Data" <- w56
                }
                n253 = VISA Close(VISA resource name=w53, error in (no error)=w52) -> (error out=w26:errorcluster)
                n254 = call <vilib>:"DAQmx Stop Task.vi"("task/channels in"=w48, "error in"=w50) -> ("error out"=w45:errorcluster)  [unwired: 12 in, 1 out]
                n255 = call <vilib>:"DAQmx Stop Task.vi"("task/channels in"=w33, "error in"=w34) -> ("error out"=w35:errorcluster)  [unwired: 12 in, 1 out]
                n256 = call <vilib>:"DAQmx Stop Task.vi"("task/channels in"=w40, "error in"=w41) -> ("error out"=w39:errorcluster)  [unwired: 12 in, 1 out]
                n257 = Unbundle By Name(w26) -> ("status"=w27:bool)
                n258 = call <vilib>:"Simple Error Handler.vi"("error in (no error)"=w45) -> ()  [unwired: 4 in, 5 out]
                n259 = call <vilib>:"Simple Error Handler.vi"("error in (no error)"=w35) -> ()  [unwired: 4 in, 5 out]
                n260 = call <vilib>:"Simple Error Handler.vi"("error in (no error)"=w39) -> ()  [unwired: 4 in, 5 out]
                n261 = local write "Serial 2"(w27) -> ()
              }
            }
          }
          frame Error {
          }
        }
      }
      n262 = while {
        shift-right: [w662] -> w18
        shift-left: w17 -> [w663]
        tunnel: w8 -> [w664]
        shift-right: [w659] -> w13
        shift-left: w15 -> [w660]
        tunnel: w7 -> [w661]
        tunnel: w9 -> [_]
        shift-right: [w657] -> w12
        shift-left: w14 -> [w657]
        stop <- w658 stop-if-true
        n263 = event shown="[2] \"Recording\": Value Change" {
          selector: _ -> [_ _ _ _]
          dyn-events: _ -> [_ _ _ _]
          timeout: _ -> [_ _ _ _]
          tunnel: w664 -> [_ w672 _ _]
          tunnel: w663 -> [_ w671 _ _]
          tunnel: [_ w669 _ _] -> w662
          tunnel: w661 -> [_ w668 _ _]
          tunnel: w660 -> [_ w667 _ _]
          tunnel: [_ w665 _ _] -> w659
          tunnel: [_ _ _ "stop"] -> w656
          event Timeout {
            n264 = event-data() -> ()  [unwired: 1 in, 2 out]
          }
          event "OpenCam": Value Change {
            n265 = event-data() -> ()  [unwired: 1 in, 1 out]
            n266 = Enqueue Element(queue=w672, element=enum16{"OpenCam"}."OpenCam" ("Enum"), error in (no error)=w671) -> (error out=w669:errorcluster)  [unwired: 1 in, 2 out]
            n267 = Enqueue Element(queue=w668, element=enum16{"PosSig"}."PosSig" ("Enum"), error in (no error)=w667) -> (error out=w665:errorcluster)  [unwired: 1 in, 2 out]
          }
          event "Recording": Value Change {
            n268 = event-data() -> ()  [unwired: 1 in, 5 out]
            n269 = case shown="True" "Recording" {
              frame False {
                n270 = property on="Avi Refnum" class="TypRef (strict)"() -> ("Value"=w675:T1)  [unwired: 2 in, 2 out]
                n271 = call "IMAQ AVI Close"("Avi Refnum"=w675) -> ("error out"=w674:errorcluster)  [unwired: 10 in]
                n272 = call <vilib>:"General Error Handler.vi"("error in (no error)"=w674) -> ()  [unwired: 2 in, 13 out]
              }
              frame True {
                n273 = stacked-sequence {
                  frame #0 {
                    n274 = local read "Frame Rate"() -> (w681:dbl)
                    n275 = call "File Dialog"("pattern (all files)"="*.avi") -> ("selected path"=w679:path)  [unwired: 11 in, 3 out]
                    "Rec File Path:" <- w679
                    n276 = call "IMAQ AVI Create"("Compression Filter"="Codec:", "Frames Per Second"=w681, "AVI Path"=w679) -> ("Avi Refnum"=→"Avi Refnum":T1)  [unwired: 7 in, 1 out]
                    n277 = property on="OpenCam" class="Bool (strict)"("DisabledEnum"=T5."Disabled and Grayed Out" ("Disabled")) -> ()  [unwired: 2 in, 2 out]
                  }
                  frame #1 {
                    n278 = local read "Rec File Path:"() -> (w684:path)
                    n279 = Strip Path(path=w684) -> (stripped path=w692:path, name=w693:string)
                    n280 = Strip Path(path=w684) -> (stripped path=w689:path, name=w688:string)
                    n281 = Search and Replace String(input string=w693, search string=".avi", replace string="_VT.csv" ("replace string (\"\")")) -> (result string=w696:string)  [unwired: 5 in, 3 out]
                    n282 = Search and Replace String(input string=w688, search string=".avi", replace string="_GT.csv" ("replace string (\"\")")) -> (result string=w685:string)  [unwired: 5 in, 3 out]
                    n283 = Build Path(base path=w692, name or relative path=w696) -> (appended path=w691:path)
                    n284 = Build Path(base path=w689, name or relative path=w685) -> (appended path=w682:path)
                    n285 = call-poly <vilib>:"Write To Spreadsheet File.vi"("delimiter (\\t)"="," ("delimiter (\\t)"), "file path (dialog if empty)"=w691) -> ()  [unwired: 6 in, 1 out]
                    n286 = call-poly <vilib>:"Write To Spreadsheet File.vi"("delimiter (\\t)"="," ("delimiter (\\t)"), "file path (dialog if empty)"=w682) -> ()  [unwired: 6 in, 1 out]
                  }
                  frame #2 {
                    n287 = Get Date/Time In Seconds() -> (seconds since 1Jan1904=→"Start RecTime":timestamp)
                    "Frame Num" <- 0.0 ("Frame Num")
                    "Elapsed Time" <- 0.0 ("Elapsed Time")
                  }
                }
              }
            }
          }
          event "stop": Value Change {
            n288 = event-data() -> ()  [unwired: 1 in, 5 out]
          }
        }
        n289 = Compound Arithmetic op=OR(w656) -> (w658:bool)
      }
      n290 = property on="Tab Control" class="TabCtl (strict)"("DisabledEnum"=T5."Disabled and Grayed Out" ("Disabled")) -> ()  [unwired: 2 in, 2 out]
      n291 = Release Queue(queue=w8, error in (no error)=w18) -> ()  [unwired: 1 in, 3 out]
      n292 = Release Queue(queue=w7, error in (no error)=w13) -> ()  [unwired: 1 in, 3 out]
      n293 = Release Queue(queue=w9, error in (no error)=w12) -> ()  [unwired: 1 in, 3 out]
      n294 = while {
        tunnel: w8 -> [w523]
        stop <- w521 stop-if-true
        n295 = Dequeue Element(queue=w523) -> (element=w520:enum16{"OpenCam"}, error out=w522:errorcluster)  [unwired: 2 in, 2 out]
        n296 = case shown="No Error" w522 {
          tunnel: [_ TRUE] -> w521
          tunnel: w520 -> [w524 _]
          frame No Error {
            n297 = case shown="\"OpenCam\", Default" w524 {
              frame "OpenCam", Default {
                w533 = u32 0 ("BufferInterval")
                n298 = local write "check"(FALSE ("check")) -> ()
                n299 = call <vilib>:"IMAQdx Open Camera.vi"("Session In"="Camera Name:") -> ("error out"=w541:errorcluster, "Session Out"=w540:T2)  [unwired: 2 in, 7 out]
                n300 = call "IMAQ Create"("Image Name"="Camera Name:") -> ("New Image"=w530:T4)  [unwired: 3 in, 2 out]
                n301 = call <vilib>:"IMAQdx Configure Grab.vi"("error in"=w541, "Session In"=w540) -> ("error out"=w538:errorcluster, "Session Out"=w539:T2)  [unwired: 8 out]
                n302 = call <vilib>:"IMAQdx Enumerate Attributes.vi"("Visibility"=IMAQdx_Attribute_Visibility."Simple", "Root"="CameraAttributes", "error in"=w538, "Session In"=w539) -> ("error out"=w531:errorcluster, "Attribute Information Array"=w535:T10, "Session Out"=w532:T2)  [unwired: 5 out]
                n303 = for {
                  tunnel: w535 -> [w542] mode=indexing
                  tunnel: [w543] -> w534 mode=indexing
                  n304 = Unbundle By Name(w542) -> ("Attribute Name"=w543:string)
                  n305 = Unbundle By Name(w542) -> ()  [unwired: 1 out]
                }
                n306 = property on="Attribute Name" class="Ring (strict)"("Strings []"=w534, "Value"=w533) -> ()  [unwired: 2 in, 2 out]
                n307 = while {
                  shift-right: ["Attribute Name"] -> _
                  shift-left: w533 -> [w559]
                  tunnel: [w557] -> w527
                  tunnel: [w556] -> w528
                  tunnel: w532 -> [w555]
                  tunnel: w531 -> [w554]
                  tunnel: w530 -> [w553]
                  stop <- w549 stop-if-true
                  n308 = local read "Rec File Path:"() -> (w560:path)
                  n309 = stacked-sequence {
                    tunnel: w554 -> [w567 w589 w609]
                    tunnel: w555 -> [w568 w588 w608]
                    tunnel: w559 -> [w571 _ _]
                    tunnel: "Attribute Name" -> [w570 _ _]
                    tunnel: [_ _ w607] -> w557
                    tunnel: [_ _ w606] -> w556
                    tunnel: w553 -> [_ _ w603]
                    tunnel: [_ _ w600] -> w552
                    frame #0 {
                      n310 = Not Equal?(x=w570, y=w571) -> (x != y?=w569:bool)
                      n311 = First Call?() -> (First Call?: T/F=w565:bool)
                      n312 = Or(x=w569, y=w565) -> (x .or. y?=w566:bool)
                      n313 = case shown="True" w566 {
                        tunnel: w568 -> [_ w574]
                        tunnel: w567 -> [_ w573]
                        frame False {
                        }
                        frame True {
                          n314 = property on="Attribute Name" class="Ring (strict)"() -> ("Ring Text.Text"=w579:string)  [unwired: 2 in, 2 out]
                          n315 = property class="IMAQdx"(reference=w574, error in=w573, "Camera Attributes:Active Attribute"=w579) -> (error out=w572:errorcluster, "Camera Attributes:Is Readable"=w578:bool, "Camera Attributes:Is Writable"=w587:bool, "Camera Attributes:Value:String"=w577:string)  [unwired: 1 out]
                          n316 = And(x=w578, y=w587) -> (x .and. y?=w583:bool)
                          n317 = call <vilib>:"Clear Errors.vi"("error in (no error)"=w572) -> ()  [unwired: 6 in, 1 out]
                          n318 = Select(t=0, s=w583, f=2) -> (s? t:f=w582:i32)
                          n319 = Select(t=0, s=w587, f=2) -> (s? t:f=w586:i32)
                          n320 = Select(t=w577, s=w578, f="") -> (s? t:f=w576:string)
                          n321 = property on="Attribute Value" class="Str"("Disabled"=w582) -> ()  [unwired: 2 in, 2 out]
                          n322 = property on="Set" class="Bool"("Disabled"=w586) -> ()  [unwired: 2 in, 2 out]
                          n323 = property on="Attribute Value" class="Str"("Value"=w576) -> ()  [unwired: 2 in, 2 out]
                        }
                      }
                    }
                    frame #1 {
                      n324 = case shown="True" "Set" {
                        tunnel: w589 -> [_ w592]
                        tunnel: w588 -> [_ w591]
                        frame False {
                        }
                        frame True {
                          n325 = property on="Attribute Value" class="Str"() -> ("Value"=w594:string)  [unwired: 2 in, 2 out]
                          n326 = property on="Attribute Name" class="Ring (strict)"() -> ("Ring Text.Text"=w593:string)  [unwired: 2 in, 2 out]
                          n327 = property class="IMAQdx"(reference=w591, error in=w592, "Camera Attributes:Active Attribute"=w593, "Camera Attributes:Value:String"=w594) -> (error out=w596:errorcluster, "Camera Attributes:Value:String"=w595:string)  [unwired: 1 out]
                          n328 = property on="Attribute Value" class="Str"("Value"=w595) -> ()  [unwired: 2 in, 2 out]
                          n329 = call <vilib>:"Simple Error Handler.vi"("error in (no error)"=w596) -> ()  [unwired: 1 in, 8 out]
                        }
                      }
                    }
                    frame #2 {
                      n330 = call <vilib>:"IMAQdx Grab.vi"("error in"=w609, "Image In"=w603, "Session In"=w608) -> ("error out"=w606:errorcluster, "Buffer Number Out"=w610:u32, "Image Out"=w604:T4, "Session Out"=w607:T2)  [unwired: 1 in, 4 out]
                      n331 = case shown="3, Default" "Image Flip" {
                        tunnel: w604 -> [w620 w626 w629 w631]
                        tunnel: [w619 w625 w627 w631] -> w600
                        tunnel: "Image Flip" -> [w622 w624 w628 _]
                        tunnel: w603 -> [w621 w623 w630 _]
                        frame 0 {
                          n332 = call "IMAQ Symmetry"("Type of Symmetry"=w622, "Image Dst"=w621, "Image Src"=w620) -> ("Image Dst Out"=w619:T4)  [unwired: 2 in, 1 out]
                        }
                        frame 1 {
                          n333 = call "IMAQ Symmetry"("Type of Symmetry"=w624, "Image Dst"=w623, "Image Src"=w626) -> ("Image Dst Out"=w625:T4)  [unwired: 2 in, 1 out]
                        }
                        frame 2 {
                          n334 = call "IMAQ Symmetry"("Type of Symmetry"=w628, "Image Dst"=w630, "Image Src"=w629) -> ("Image Dst Out"=w627:T4)  [unwired: 2 in, 1 out]
                        }
                        frame 3, Default {
                        }
                      }
                      n335 = call "CalculateFPS.vi"("buffer number"=w610) -> ("processed FPS"=→"Frame Rate":dbl)  [unwired: 2 out]
                      n336 = case shown="\"Alignment\", Default" "Tab Control" {
                        tunnel: w600 -> [w612 w618]
                        tunnel: "BCGT" -> [w617 _]
                        tunnel: [w612 w618] -> w598
                        tunnel: [w611 _] -> w597
                        frame "Alignment", Default {
                          n337 = call "AlignProc.vi"("BCGT"=w617, "Img_In"=w612) -> ("Distances"=→"Distances":sgl[], "Number of Particles"=→"Number of Particles":i32, "Boolean"=→"Alignment":bool, "Image Out"=w611:T4, "Array"=→"Array":cluster{"Numeric":dbl, "Numeric":dbl}[])  [unwired: 5 in]
                        }
                        frame "Rotator" {
                        }
                      }
                      "Image 2" <- w597
                      "Image" <- w598
                      n338 = property on="Image" class="ImageControl" props=["Value"]() -> ()  [unwired: 2 in, 3 out]
                    }
                  }
                  n339 = property on="Recording" class="Bool (strict)"("DisabledEnum"=T5."Enabled" ("Disabled")) -> ()  [unwired: 2 in, 2 out]
                  n340 = local read "Recording"() -> (w548:bool)
                  n341 = Not Equal?(x=w560, y=path "") -> (x != y?=w562:bool)
                  n342 = And(x=w562, y=w548) -> (x .and. y?=w561:bool)
                  n343 = case shown="False" w561 {
                    tunnel: w552 -> [_ w635]
                    tunnel: w560 -> [_ w634]
                    frame False {
                      w633 = 0.0 ("Frame Num")
                      n344 = property on="OpenCam" class="Bool (strict)"("DisabledEnum"=T5."Enabled" ("Disabled")) -> ()  [unwired: 2 in, 2 out]
                      n345 = local write "Frame Num"(w633) -> ()
                      n346 = local write "Elapsed Time"(w633) -> ()
                    }
                    frame True {
                      n347 = stacked-sequence {
                        tunnel: w635 -> [w638 _]
                        tunnel: w634 -> [_ w642]
                        frame #0 {
                          n348 = local read "Avi Refnum"() -> (w636:T1)
                          n349 = call "IMAQ AVI Write Frame"("Image"=w638, "Avi Refnum"=w636) -> ("error out"=w637:errorcluster)  [unwired: 8 in, 1 out]
                          n350 = call <vilib>:"Clear Errors.vi"("error in (no error)"=w637) -> ()  [unwired: 6 in, 1 out]
                        }
                        frame #1 {
                          n351 = local read "Start RecTime"() -> (w653:timestamp)
                          n352 = local read "Frame Num"() -> (w639:dbl)
                          n353 = Strip Path(path=w642) -> (stripped path=w644:path, name=w645:string)
                          n354 = Search and Replace String(input string=w645, search string=".avi", replace string="_VT.csv" ("replace string (\"\")")) -> (result string=w648:string)  [unwired: 5 in, 3 out]
                          n355 = Get Date/Time In Seconds() -> (seconds since 1Jan1904=w652:timestamp)
                          n356 = Build Path(base path=w644, name or relative path=w648) -> (appended path=w643:path)
                          n357 = Increment(x=w639) -> (x+1=w654:dbl)
                          n358 = Subtract(x=w652, y=w653) -> (x-y=w641:dbl)
                          n359 = local write "Frame Num"(w654) -> ()
                          n360 = local write "Elapsed Time"(w641) -> ()
                          n361 = Build Array(w641, w639) -> (w640:dbl[])
                          n362 = call-poly <vilib>:"Write To Spreadsheet File.vi"("delimiter (\\t)"="," ("delimiter (\\t)"), "transpose? (no:F)"=FALSE, "append to file? (new file:F)"=TRUE, "1D data"=w640, "file path (dialog if empty)"=w643) -> ()  [unwired: 3 in, 1 out]
                        }
                      }
                    }
                  }
                  n363 = Unbundle By Name(w556) -> ("status"=w551:bool)
                  n364 = Not(x="OpenCam") -> (.not. x?=w550:bool)
                  n365 = Select(t=T5."Enabled" ("Disabled"), s="OpenCam", f=T5."Disabled and Grayed Out" ("Disabled")) -> (s? t:f=w547:T5)
                  n366 = Or(x=w550, y=w551) -> (x .or. y?=w549:bool)
                  n367 = property on="Tab Control" class="TabCtl (strict)"("DisabledEnum"=w547) -> ()  [unwired: 2 in, 2 out]
                }
                n368 = call <vilib>:"IMAQdx Close Camera.vi"("error in"=w528, "Session In"=w527) -> ("error out"=w526:errorcluster)  [unwired: 9 out]
                n369 = call <vilib>:"General Error Handler.vi"("error in (no error)"=w526) -> ()  [unwired: 2 in, 13 out]
              }
            }
          }
          frame Error {
          }
        }
      }
    }
  }
